vi "Make_component_similarity_map.vi"(11 "Odour component data":T1) -> (3 "input cluster":cluster{"MDS1":dbl[], "MDS2":dbl[]})   [LabVIEW 2016]
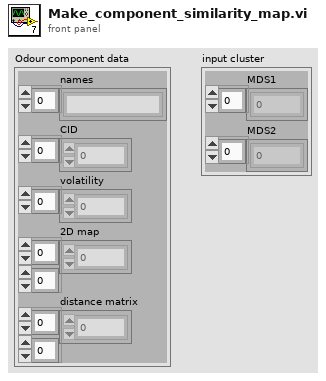
[diagram p1: front panel]
types:
  T1 = cluster{"names":string[], "CID":i32[], "volatility":dbl[], "2D map":dbl[][], "distance matrix":dbl[][]}
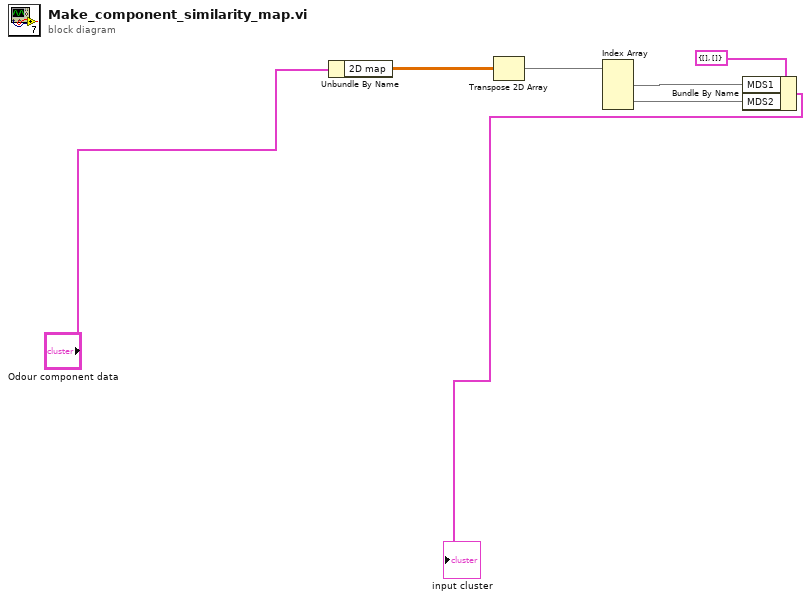
[diagram p0: block diagram]
diagram:
  n1 = Unbundle By Name("Odour component data") -> ("2D map"=w3:dbl[][])
  n2 = Transpose 2D Array(2D array=w3) -> (transposed array=w4:dbl[][])
  n3 = Index Array(array=w4) -> (element #1=w5:dbl[], element #2=w6:dbl[])  [unwired: 4 in]
  n4 = Bundle By Name(cluster=cluster{"MDS1":dbl[], "MDS2":dbl[]} {"MDS1"=[], "MDS2"=[]} ("input cluster"), "MDS1"=w5, "MDS2"=w6) -> (→"input cluster":cluster{"MDS1":dbl[], "MDS2":dbl[]})
